vi "Start Testing.vi"(8 "error in (no error)":errorcluster, 9 "Test Settings":T1, 10 "Model in":refnum<class "Model.lvclass">, 11 "Wait For User Input State in":refnum<class "Wait For User Input State.lvclass">) -> (0 "error out":errorcluster, 2 "Model out":refnum<class "Model.lvclass">, 3 "Wait For User Input State out":refnum<class "Wait For User Input State.lvclass">)   [LabVIEW 2016, in "Wait For User Input State.lvclass"]
uses:
  Wait For User Input State.lvclass
  Model/Model/Model.lvclass
  Typedefs/TestSettings.ctl
  Typedefs/StateTypes.ctl
  common_rt_hpilc/HPILCFactory/HPILCFactory.lvclass
  Model/Model/Model.lvclass/Model.ctl
  Typedefs/HPMT_Typedefs.lvlib
  Model/Boot Loader/Boot Loader.lvclass
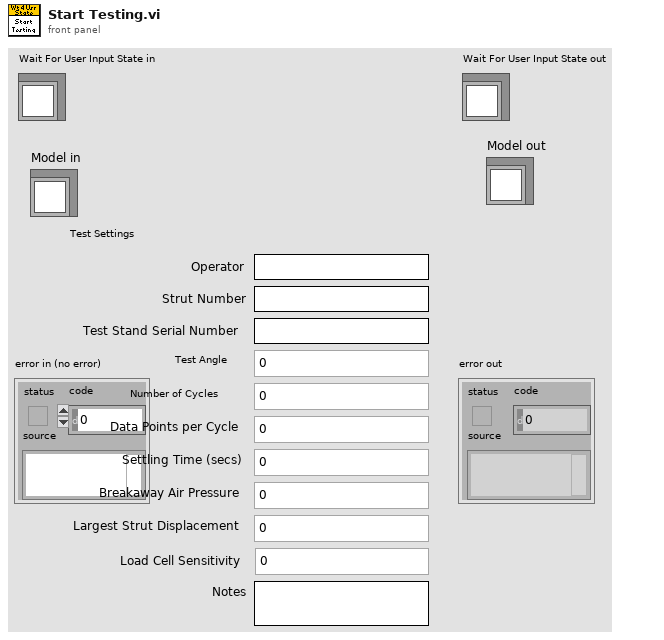
[diagram p1: front panel]
types:
  T1 = typedef "HPMT_Typedefs.lvlib/TestSettings.ctl" = cluster{"Operator":string, "Strut Number":string, "Test Stand Serial Number":string, "Notes":string, "Test Angle":u16, "Number of Cycles":u16, "Data Points per Cycle":u16, "Settling Time (secs)":u16, "Breakaway Air Pressure":u16, "Largest Strut Displacement":dbl, "Load Cell Sensitivity":dbl}
  T2 = typedef "HPMT_Typedefs.lvlib/StateTypes.ctl" = enum16{"Offline State", "Fault State", "Standby State", "Disabled State", "Enabled State", "Wait For User Input State", "Test Actuator State", "Manual State"}
  T3 = typedef "RTHPILC.lvlib/HPSettings.ctl" = cluster{"ILCSettings":T4, "ID":i16, "ReferencePosition":i32}
  T4 = typedef "RTILC.lvlib/ILCSettings.ctl" = cluster{"Subnet":u8, "Address":u8}
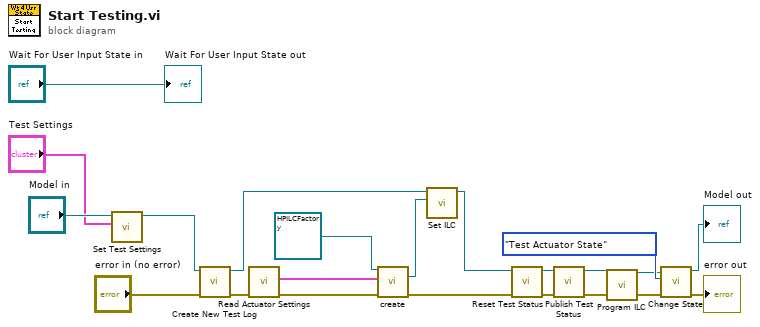
[diagram p0: block diagram]
diagram:
  n1 = call "Set Test Settings.vi"("Test Settings"="Test Settings", "Model in"="Model in") -> ("Model out"=w16:refnum<class "Model.lvclass">)  [unwired: 9 in]
  n2 = call "Create New Test Log.vi"("error in (no error)"="error in (no error)", "Model in"=w16) -> ("error out"=w14:errorcluster, "Model out"=w12:refnum<class "Model.lvclass">)  [unwired: 8 in]
  n3 = call "Read Actuator Settings.vi"("error in (no error)"=w14) -> ("error out"=w13:errorcluster, "HPSettings"=w5:T3)  [unwired: 8 in, 1 out]
  n4 = call "create.vi"("HPILCFactory in"=refnum<class "HPILCFactory.lvclass"> refnum ("RTHPILC.lvlib:HPILCFactory.lvclass"), "HPSettings"=w5, "error in (no error)"=w13) -> ("HPILC"=w6:refnum<class "HPILC.lvclass">, "error out"=w10:errorcluster)  [unwired: 10 in, 1 out]
  n5 = call "Set ILC.vi"("HPILC"=w6, "Model in"=w12) -> ("Model out"=w11:refnum<class "Model.lvclass">)  [unwired: 9 in]
  n6 = call "Reset Test Status.vi"("error in (no error)"=w10, "Model in"=w11) -> ("error out"=w8:errorcluster, "Model out"=w9:refnum<class "Model.lvclass">)  [unwired: 8 in]
  n7 = call "Publish Test Status.vi"("error in (no error)"=w8, "Model in"=w9) -> ("error out"=w1:errorcluster, "Model out"=w4:refnum<class "Model.lvclass">)  [unwired: 8 in]
  n8 = call "Program ILC.vi"("Model in"=w4, "error in (no error)"=w1) -> ("Model out"=w3:refnum<class "Model.lvclass">, "error out"=w2:errorcluster)  [unwired: 12 in]
  n9 = call "Change State.vi"("error in (no error)"=w2, "State Types"=StateTypes."Test Actuator State" ("State:"), "Model in"=w3) -> ("error out"=→"error out":errorcluster, "Model out"=→"Model out":refnum<class "Model.lvclass">)  [unwired: 7 in]
  "Wait For User Input State out" <- "Wait For User Input State in"
